vi "PV HLT5xx Flowlimit low high.vi"(0 "VISA session":refnum<visa-resource-name>, 1 "Adress of unit":u16=1 min=1 max=999 step=1, 5 "Parameter":u16(ring) items=[" Flow limit low", " Flow limit high"], 7 "Parameter\nread only<->describe":bool, 9 "Flow limit low":u16=10 min=1 max=40 step=1, 11 "error in (no error)":errorcluster, 12 "Flow limit high":u16=50 min=10 max=50 step=1) -> (4 "dup VISA session":refnum<visa-resource-name>, 6 "response (data)":string, 15 "error out":errorcluster)   [LabVIEW 2016, in "Pfeiffer Vacuum.lvlib"]
doc: "There are 2 parameters available, only one of which can be enabled at a time. \n\n0 - Flow limit low - (default) Para 664\n1 - Flow limit high - Para 665\n\nNote: The 2 controls down of this one will set the appropriate values for the selected parameter. Any settings for an parameter that is not selected will be ignored. If a value is out of range, it will be changed to either the upper or the lower limit of the range."
uses:
  Pfeiffer Vacuum.lvlib
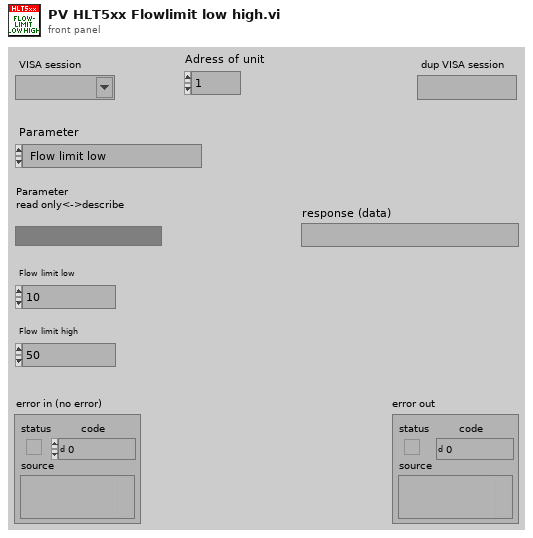
[diagram p1: front panel]
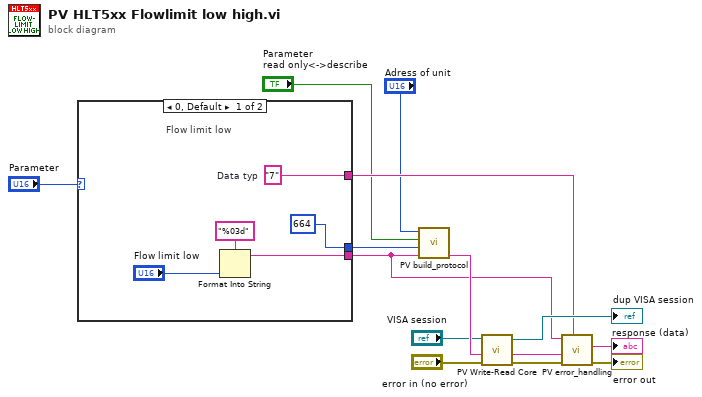
[diagram p0: block diagram]
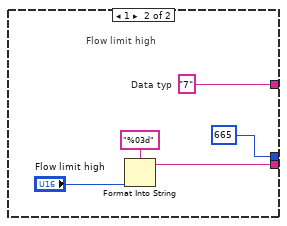
[diagram p2: hidden frame]
diagram:
  n1 = case shown="0, Default" "Parameter" {
    tunnel: [u16 664 ("Parameter-number") u16 665 ("Parameter-number")] -> w14
    tunnel: [w16 w21] -> w9
    tunnel: [w19 w24] -> w8
    frame 0, Default {
      w19 = "7"  # Data typ
      # "Flow limit low"
      n2 = Format Into String(format string="%03d" ("Format-String"), "Flow limit low") -> (resulting string=w16:string)  [unwired: 2 in, 1 out]
    }
    frame 1 {
      w24 = "7"  # Data typ
      # "Flow limit high"
      n3 = Format Into String(format string="%03d" ("Format-String"), "Flow limit high") -> (resulting string=w21:string)  [unwired: 2 in, 1 out]
    }
  }
  n4 = call "PV build_protocol.vi"("Data"=w9, "Parameter-number"=w14, "parameter\nread<->describe"="Parameter\nread only<->describe", "Adress"="Adress of unit") -> ("output"=w13:string)  [unwired: 3 in]
  n5 = call "PV Write-Read Core.vi"("error in"="error in (no error)", "Write data in"=w13, "VISA session"="VISA session") -> ("error out"=w11:errorcluster, "response (data) out"=w12:string, "dup VISA session"=→"dup VISA session":refnum<visa-resource-name>)  [unwired: 2 in]
  n6 = call "PV error_handling.vi"("Data Typ in"=w8, "error in"=w11, "response (data) in"=w12, "data in"=w9) -> ("error out"=→"error out":errorcluster, "Data out"=→"response (data)":string)  [unwired: 5 in, 1 out]
